vi "PathPlanner_Cmd_FindFollowHolonomicPathSimpleExecute.vi"(5 "PathPlanner_Cmd_FollowHolConfig":T13={"HOLONOMIC_CTRL_PACK_TUNING"={"X PID Tuning"={"Kp"=0.0, "Ki"=0.0, "Kd"=0.0, "MaximumIntegral"=9.9e+30, "MinimumIntegral"=-9.9e+30, "IntegralZone"=9.9e+30}, "Y PID Tuning"={"Kp"=0.0, "Ki"=0.0, "Kd"=0.0, "MaximumIntegral"=9.9e+30, "MinimumIntegral"=-9.9e+30, "IntegralZone"=9.9e+30}, "thetaProfiledPID_CTRL"={"Controller"={"Kp"=0.0, "Ki"=0.0, "Kd"=0.0, "Period"=0.0, "Max_Integral"=1.0, "Min_Integral"=-1.0, "Max_Input"=0.0, "Min_Input"=0.0, "Continuous"=FALSE, "PositionError"=0.0, "VelocityError"=0.0, "PrevError"=0.0, "Total_Integral"=0.0, "PositionTolerance"=0.05, "VelocityTolerance"=9.99e+35, "SetPoint"=0.0, "Kf"=0.0, "Prev_Deriv"=0.0, "Prev_Deriv 2"=0.0, "DerivativeFilter"=FALSE, "Min_Output"=-9.99e+35, "Max_Output"=9.9e+35, "Prev_F_P"=0.0, "Prev_F_P_2"=0.0, "AntiWindupActive"=FALSE, "Measurement"=0.0, "IntegralZone"=9.9e+30}, "Goal"={"Position"=0.0, "Velocity"=0.0}, "Setpoint"={"Position"=0.0, "Velocity"=0.0}, "Constraint"={"MaxVelocity"=0.0, "MaxAcceleration"=0.0}}}, "Max Wheel Speed M/S"=0.0, "Tolerance SI"={"TRANSLATION"={"X"=0.04, "Y"=0.04}, "ROTATION"={"VALUE"=0.034906585039887, "COS"=0.999390827019096, "SIN"=0.034899496702501}}, "Drive Base Radius M"=0.0, "ControlPastEnd_Sec"=3.0, "ReplanningConfig"={"enableInitialReplanning"=FALSE, "enableDynamicReplanning"=FALSE, "dynamicReplanningTotalErrorThreshold"=0.0, "dynamicReplanningErrorSpikeThreshold"=0.0}, "Period_Sec"=0.02, "Trigger Events"=TRUE} {"Tolerance SI"."ROTATION"."SIN" format="%13.4f"; "Tolerance SI"."ROTATION"."COS" format="%13.4f"; "Tolerance SI"."ROTATION"."VALUE" format="%13.4f"; "Tolerance SI"."TRANSLATION"."Y" format="%14.3f"; "Tolerance SI"."TRANSLATION"."X" format="%14.3f"; "HOLONOMIC_CTRL_PACK_TUNING"."thetaProfiledPID_CTRL"."Constraint"."MaxAcceleration" format="%16_6e"; "HOLONOMIC_CTRL_PACK_TUNING"."thetaProfiledPID_CTRL"."Constraint"."MaxVelocity" format="%16_6e"; "HOLONOMIC_CTRL_PACK_TUNING"."thetaProfiledPID_CTRL"."Setpoint"."Velocity" format="%16_6e"; "HOLONOMIC_CTRL_PACK_TUNING"."thetaProfiledPID_CTRL"."Setpoint"."Position" format="%16_6e"; "HOLONOMIC_CTRL_PACK_TUNING"."thetaProfiledPID_CTRL"."Goal"."Velocity" format="%16_6e"; "HOLONOMIC_CTRL_PACK_TUNING"."thetaProfiledPID_CTRL"."Goal"."Position" format="%16_6e"; "HOLONOMIC_CTRL_PACK_TUNING"."thetaProfiledPID_CTRL"."Controller"."IntegralZone" format="%16_6e"; "HOLONOMIC_CTRL_PACK_TUNING"."thetaProfiledPID_CTRL"."Controller"."Measurement" format="%16_6e"; "HOLONOMIC_CTRL_PACK_TUNING"."thetaProfiledPID_CTRL"."Controller"."Prev_F_P_2" format="%16_6e"; "HOLONOMIC_CTRL_PACK_TUNING"."thetaProfiledPID_CTRL"."Controller"."Prev_F_P" format="%16_6e"; "HOLONOMIC_CTRL_PACK_TUNING"."thetaProfiledPID_CTRL"."Controller"."Max_Output" format="%16_6e"; "HOLONOMIC_CTRL_PACK_TUNING"."thetaProfiledPID_CTRL"."Controller"."Min_Output" format="%16_6e"; "HOLONOMIC_CTRL_PACK_TUNING"."thetaProfiledPID_CTRL"."Controller"."Prev_Deriv 2" format="%16_6e"; "HOLONOMIC_CTRL_PACK_TUNING"."thetaProfiledPID_CTRL"."Controller"."Prev_Deriv" format="%16_6e"; "HOLONOMIC_CTRL_PACK_TUNING"."thetaProfiledPID_CTRL"."Controller"."Kf" format="%16_6e"; "HOLONOMIC_CTRL_PACK_TUNING"."thetaProfiledPID_CTRL"."Controller"."SetPoint" format="%16_6e"; "HOLONOMIC_CTRL_PACK_TUNING"."thetaProfiledPID_CTRL"."Controller"."VelocityTolerance" format="%16_6e"; "HOLONOMIC_CTRL_PACK_TUNING"."thetaProfiledPID_CTRL"."Controller"."PositionTolerance" format="%16_6e"; "HOLONOMIC_CTRL_PACK_TUNING"."thetaProfiledPID_CTRL"."Controller"."Total_Integral" format="%16_6e"; "HOLONOMIC_CTRL_PACK_TUNING"."thetaProfiledPID_CTRL"."Controller"."PrevError" format="%16_6e"; "HOLONOMIC_CTRL_PACK_TUNING"."thetaProfiledPID_CTRL"."Controller"."VelocityError" format="%16_6e"; "HOLONOMIC_CTRL_PACK_TUNING"."thetaProfiledPID_CTRL"."Controller"."PositionError" format="%16_6e"; "HOLONOMIC_CTRL_PACK_TUNING"."thetaProfiledPID_CTRL"."Controller"."Min_Input" format="%16_6e"; "HOLONOMIC_CTRL_PACK_TUNING"."thetaProfiledPID_CTRL"."Controller"."Max_Input" format="%16_6e"; "HOLONOMIC_CTRL_PACK_TUNING"."thetaProfiledPID_CTRL"."Controller"."Min_Integral" format="%16_6e"; "HOLONOMIC_CTRL_PACK_TUNING"."thetaProfiledPID_CTRL"."Controller"."Max_Integral" format="%16_6e"; "HOLONOMIC_CTRL_PACK_TUNING"."thetaProfiledPID_CTRL"."Controller"."Period" format="%16_6e"; "HOLONOMIC_CTRL_PACK_TUNING"."thetaProfiledPID_CTRL"."Controller"."Kd" format="%16_6e"; "HOLONOMIC_CTRL_PACK_TUNING"."thetaProfiledPID_CTRL"."Controller"."Ki" format="%16_6e"; "HOLONOMIC_CTRL_PACK_TUNING"."thetaProfiledPID_CTRL"."Controller"."Kp" format="%16_6e"}, 6 "PassthroughTime_SEC":dbl=-1.0, 7 "PathPlanner_Cmd_FindConfig":T1={"Goal Position"={"X"=0.0, "Y"=0.0}, "GoalEndState"={"VelocityMPS"=0.0, "Rotation"={"VALUE"=0.0, "COS"=1.0, "SIN"=0.0}}, "PathPlannerPathConstraints"={"MaxVelocityMps;"=0.0, "MaxAccelerationMpsSq;"=0.0, "MaxAngularVelRadPsEc;"=0.0, "MaxAngularAccRadPSecSq"=0.0, "Exists"=FALSE, "Unlimited"=FALSE, "NominalVoltageVolts"=12.0}, "Rotation Delay Distance M"=0.0} {"GoalEndState"."Rotation"."SIN" format="%13.4f"; "GoalEndState"."Rotation"."COS" format="%13.4f"; "GoalEndState"."Rotation"."VALUE" format="%13.4f"; "Goal Position"."Y" step=0.25 format="%14.3f"; "Goal Position"."X" format="%14.3f"}, 8 "Enabled":bool=TRUE, 9 "Reset":bool, 10 "CurrentChassisSpeeds":T6 {"vOmega" format="%10.3f"; "vY" format="%10.3f"; "vX" format="%10.3f"}, 11 "Current Pose SI":T8={"TRANSLATION"={"X"=0.0, "Y"=0.0}, "ROTATION"={"VALUE"=0.0, "COS"=1.0, "SIN"=0.0}} {"ROTATION"."SIN" format="%13.4f"; "ROTATION"."COS" format="%13.4f"; "ROTATION"."VALUE" format="%13.4f"; "TRANSLATION"."Y" format="%14.3f"; "TRANSLATION"."X" format="%14.3f"}) -> (0 "Position Error M":dbl, 1 "Complete":bool, 2 "At Reference":bool, 3 "calcChassisSpeed":T6 {"vOmega" format="%10.3f"; "vY" format="%10.3f"; "vX" format="%10.3f"}, 4 "outHOLONOMIC_DRV_CTRL":T7={"poseTolerance"={"TRANSLATION"={"X"=0.0, "Y"=0.0}, "ROTATION"={"VALUE"=0.0, "COS"=1.0, "SIN"=0.0}}, "poseError"={"TRANSLATION"={"X"=0.0, "Y"=0.0}, "ROTATION"={"VALUE"=0.0, "COS"=1.0, "SIN"=0.0}}, "Enabled"=TRUE, "PID_xCtrl"={"Kp"=0.0, "Ki"=0.0, "Kd"=0.0, "Period"=0.0, "Max_Integral"=1.0, "Min_Integral"=-1.0, "Max_Input"=0.0, "Min_Input"=0.0, "Continuous"=FALSE, "PositionError"=0.0, "VelocityError"=0.0, "PrevError"=0.0, "Total_Integral"=0.0, "PositionTolerance"=0.05, "VelocityTolerance"=9.99e+35, "SetPoint"=0.0, "Kf"=0.0, "Prev_Deriv"=0.0, "Prev_Deriv 2"=0.0, "DerivativeFilter"=FALSE, "Min_Output"=-9.99e+35, "Max_Output"=9.9e+35, "Prev_F_P"=0.0, "Prev_F_P_2"=0.0, "AntiWindupActive"=FALSE, "Measurement"=0.0, "IntegralZone"=9.9e+30}, "PID_yCtrl"={"Kp"=0.0, "Ki"=0.0, "Kd"=0.0, "Period"=0.0, "Max_Integral"=1.0, "Min_Integral"=-1.0, "Max_Input"=0.0, "Min_Input"=0.0, "Continuous"=FALSE, "PositionError"=0.0, "VelocityError"=0.0, "PrevError"=0.0, "Total_Integral"=0.0, "PositionTolerance"=0.05, "VelocityTolerance"=9.99e+35, "SetPoint"=0.0, "Kf"=0.0, "Prev_Deriv"=0.0, "Prev_Deriv 2"=0.0, "DerivativeFilter"=FALSE, "Min_Output"=-9.99e+35, "Max_Output"=9.9e+35, "Prev_F_P"=0.0, "Prev_F_P_2"=0.0, "AntiWindupActive"=FALSE, "Measurement"=0.0, "IntegralZone"=9.9e+30}, "PROF_PID_thetaCtrl"={"Controller"={"Kp"=0.0, "Ki"=0.0, "Kd"=0.0, "Period"=0.0, "Max_Integral"=1.0, "Min_Integral"=-1.0, "Max_Input"=0.0, "Min_Input"=0.0, "Continuous"=FALSE, "PositionError"=0.0, "VelocityError"=0.0, "PrevError"=0.0, "Total_Integral"=0.0, "PositionTolerance"=0.05, "VelocityTolerance"=9.99e+35, "SetPoint"=0.0, "Kf"=0.0, "Prev_Deriv"=0.0, "Prev_Deriv 2"=0.0, "DerivativeFilter"=FALSE, "Min_Output"=-9.99e+35, "Max_Output"=9.9e+35, "Prev_F_P"=0.0, "Prev_F_P_2"=0.0, "AntiWindupActive"=FALSE, "Measurement"=0.0, "IntegralZone"=9.9e+30}, "Goal"={"Position"=0.0, "Velocity"=0.0}, "Setpoint"={"Position"=0.0, "Velocity"=0.0}, "Constraint"={"MaxVelocity"=0.0, "MaxAcceleration"=0.0}}, "RotationError"={"VALUE"=0.0, "COS"=1.0, "SIN"=0.0}, "FirstRun"=TRUE} {"RotationError"."SIN" format="%13.4f"; "RotationError"."COS" format="%13.4f"; "RotationError"."VALUE" format="%13.4f"; "PROF_PID_thetaCtrl"."Constraint"."MaxAcceleration" format="%16_6e"; "PROF_PID_thetaCtrl"."Constraint"."MaxVelocity" format="%16_6e"; "PROF_PID_thetaCtrl"."Setpoint"."Velocity" format="%16_6e"; "PROF_PID_thetaCtrl"."Setpoint"."Position" format="%16_6e"; "PROF_PID_thetaCtrl"."Goal"."Velocity" format="%16_6e"; "PROF_PID_thetaCtrl"."Goal"."Position" format="%16_6e"; "PROF_PID_thetaCtrl"."Controller"."IntegralZone" format="%16_6e"; "PROF_PID_thetaCtrl"."Controller"."Measurement" format="%16_6e"; "PROF_PID_thetaCtrl"."Controller"."Prev_F_P_2" format="%16_6e"; "PROF_PID_thetaCtrl"."Controller"."Prev_F_P" format="%16_6e"; "PROF_PID_thetaCtrl"."Controller"."Max_Output" format="%16_6e"; "PROF_PID_thetaCtrl"."Controller"."Min_Output" format="%16_6e"; "PROF_PID_thetaCtrl"."Controller"."Prev_Deriv 2" format="%16_6e"; "PROF_PID_thetaCtrl"."Controller"."Prev_Deriv" format="%16_6e"; "PROF_PID_thetaCtrl"."Controller"."Kf" format="%16_6e"; "PROF_PID_thetaCtrl"."Controller"."SetPoint" format="%16_6e"; "PROF_PID_thetaCtrl"."Controller"."VelocityTolerance" format="%16_6e"; "PROF_PID_thetaCtrl"."Controller"."PositionTolerance" format="%16_6e"; "PROF_PID_thetaCtrl"."Controller"."Total_Integral" format="%16_6e"; "PROF_PID_thetaCtrl"."Controller"."PrevError" format="%16_6e"; "PROF_PID_thetaCtrl"."Controller"."VelocityError" format="%16_6e"; "PROF_PID_thetaCtrl"."Controller"."PositionError" format="%16_6e"; "PROF_PID_thetaCtrl"."Controller"."Min_Input" format="%16_6e"; "PROF_PID_thetaCtrl"."Controller"."Max_Input" format="%16_6e"; "PROF_PID_thetaCtrl"."Controller"."Min_Integral" format="%16_6e"; "PROF_PID_thetaCtrl"."Controller"."Max_Integral" format="%16_6e"; "PROF_PID_thetaCtrl"."Controller"."Period" format="%16_6e"; "PROF_PID_thetaCtrl"."Controller"."Kd" format="%16_6e"; "PROF_PID_thetaCtrl"."Controller"."Ki" format="%16_6e"; "PROF_PID_thetaCtrl"."Controller"."Kp" format="%16_6e"; "PID_yCtrl"."IntegralZone" format="%16_6e"; "PID_yCtrl"."Measurement" format="%16_6e"; "PID_yCtrl"."Prev_F_P_2" format="%16_6e"; "PID_yCtrl"."Prev_F_P" format="%16_6e"; "PID_yCtrl"."Max_Output" format="%16_6e"; "PID_yCtrl"."Min_Output" format="%16_6e"; "PID_yCtrl"."Prev_Deriv 2" format="%16_6e"; "PID_yCtrl"."Prev_Deriv" format="%16_6e"; "PID_yCtrl"."Kf" format="%16_6e"; "PID_yCtrl"."SetPoint" format="%16_6e"; "PID_yCtrl"."VelocityTolerance" format="%16_6e"; "PID_yCtrl"."PositionTolerance" format="%16_6e"; "PID_yCtrl"."Total_Integral" format="%16_6e"; "PID_yCtrl"."PrevError" format="%16_6e"; "PID_yCtrl"."VelocityError" format="%16_6e"; "PID_yCtrl"."PositionError" format="%16_6e"; "PID_yCtrl"."Min_Input" format="%16_6e"; "PID_yCtrl"."Max_Input" format="%16_6e"; "PID_yCtrl"."Min_Integral" format="%16_6e"; "PID_yCtrl"."Max_Integral" format="%16_6e"; "PID_yCtrl"."Period" format="%16_6e"; "PID_yCtrl"."Kd" format="%16_6e"; "PID_yCtrl"."Ki" format="%16_6e"; "PID_yCtrl"."Kp" format="%16_6e"; "PID_xCtrl"."IntegralZone" format="%16_6e"; "PID_xCtrl"."Measurement" format="%16_6e"; "PID_xCtrl"."Prev_F_P_2" format="%16_6e"; "PID_xCtrl"."Prev_F_P" format="%16_6e"; "PID_xCtrl"."Max_Output" format="%16_6e"; "PID_xCtrl"."Min_Output" format="%16_6e"; "PID_xCtrl"."Prev_Deriv 2" format="%16_6e"; "PID_xCtrl"."Prev_Deriv" format="%16_6e"; "PID_xCtrl"."Kf" format="%16_6e"; "PID_xCtrl"."SetPoint" format="%16_6e"; "PID_xCtrl"."VelocityTolerance" format="%16_6e"; "PID_xCtrl"."PositionTolerance" format="%16_6e"; "PID_xCtrl"."Total_Integral" format="%16_6e"; "PID_xCtrl"."PrevError" format="%16_6e"; "PID_xCtrl"."VelocityError" format="%16_6e"; "PID_xCtrl"."PositionError" format="%16_6e"; "PID_xCtrl"."Min_Input" format="%16_6e"; "PID_xCtrl"."Max_Input" format="%16_6e"; "PID_xCtrl"."Min_Integral" format="%16_6e"; "PID_xCtrl"."Max_Integral" format="%16_6e"; "PID_xCtrl"."Period" format="%16_6e"; "PID_xCtrl"."Kd" format="%16_6e"; "PID_xCtrl"."Ki" format="%16_6e"; "PID_xCtrl"."Kp" format="%16_6e"; "poseError"."ROTATION"."SIN" format="%13.4f"; "poseError"."ROTATION"."COS" format="%13.4f"; "poseError"."ROTATION"."VALUE" format="%13.4f"; "poseError"."TRANSLATION"."Y" format="%14.3f"; "poseError"."TRANSLATION"."X" format="%14.3f"; "poseTolerance"."ROTATION"."SIN" format="%13.4f"; "poseTolerance"."ROTATION"."COS" format="%13.4f"; "poseTolerance"."ROTATION"."VALUE" format="%13.4f"; "poseTolerance"."TRANSLATION"."Y" format="%14.3f"; "poseTolerance"."TRANSLATION"."X" format="%14.3f"})   [LabVIEW 2019, in "PathPlanner24.lvlib"]
doc: "DOCUMENTATION IS NOT COMPLETE.\n\nFind and follow a path for holonomic (swerve and mecanum) drive robots using holonomic controller.\n \n \nInputs:\n - CurrentPoseSi - pose2d - The current pose calculated by odometry or pose estimation. The pose can be absolute or relative depending on what type of trajectory is being followed.\n - Reset - boolean - When TRUE the holonomic drive controller is reset. This should be set to TRUE for the first execution of a trajectory.\n - Enabled - boolean - When TRUE, closed loop control is enabled. (Optional. Default: TRUE)\n - Period - double - The loop period in seconds for this controller. (Optional. Default: 0.020)\n\nOutputs:\n - CalcChassisSpeed - cluster - The desired chassis speed in SI units.\n - AtReference - boolean - TRUE if the robots position is within the defined tolerance.\n - PositionError - pose2d - Position error in SI units. How far the robot is away from the desired trajectory position.\n - out_Holonomic_Drive_Ctrl - THe current holonomic drive controller data cluster. This is mainly for diagnostic purposes."
uses:
  PathPlanner24.lvlib
  <vilib>/Rock Robotics/WPI/ThirdParty/JAS_Junk/TrajLib/TypeDef/POSE2D.ctl
  <vilib>/Rock Robotics/WPI/ThirdParty/JAS_Junk/TrajLib/TypeDef/TRANSLATION2D.ctl
  <vilib>/Rock Robotics/WPI/ThirdParty/JAS_Junk/TrajLib/TypeDef/ROTATION2D.ctl
  TypeDef/PathPlannerCmdFollowHolConfig.ctl
  <vilib>/Rock Robotics/WPI/ThirdParty/JAS_Junk/TrajLib/TypeDef/HOLONOMIC_PACK_TUNING.ctl
  <vilib>/Rock Robotics/WPI/ThirdParty/JAS_Junk/TrajLib/TypeDef/PID_TUNING.ctl
  <vilib>/Rock Robotics/WPI/ThirdParty/JAS_Junk/TrajLib/TypeDef/PROFILED_PID_CONTROLLER.ctl
  <vilib>/Rock Robotics/WPI/ThirdParty/JAS_Junk/TrajLib/TypeDef/PID_CONTROLLER.ctl
  <vilib>/Rock Robotics/WPI/ThirdParty/JAS_Junk/TrajLib/TypeDef/TRAPEZOID_PROFILE_STATE.ctl
  <vilib>/Rock Robotics/WPI/ThirdParty/JAS_Junk/TrajLib/TypeDef/TRAPEZOID_PROFILE_CONSTRAINT.ctl
  TypeDef/PathPlannerReplanningConfig.ctl
  <vilib>/Rock Robotics/WPI/ThirdParty/JAS_Junk/TrajLib/TypeDef/HOLONOMIC_DRV_CTRL.ctl
  <vilib>/Rock Robotics/WPI/ThirdParty/JAS_Junk/TrajLib/TypeDef/CHASSIS_SPEEDS.ctl
  TypeDef/PathPlannerCmdFindConfig.ctl
  TypeDef/PathPlannerGoalEndState.ctl
  TypeDef/PathPlannerPathConstraints.ctl
  <vilib>/Rock Robotics/WPI/ThirdParty/JAS_Junk/TrajLib/Util_CalcDist.vi
  <vilib>/Rock Robotics/WPI/ThirdParty/JAS_Junk/TrajLib/Trajectory_Library.lvlib
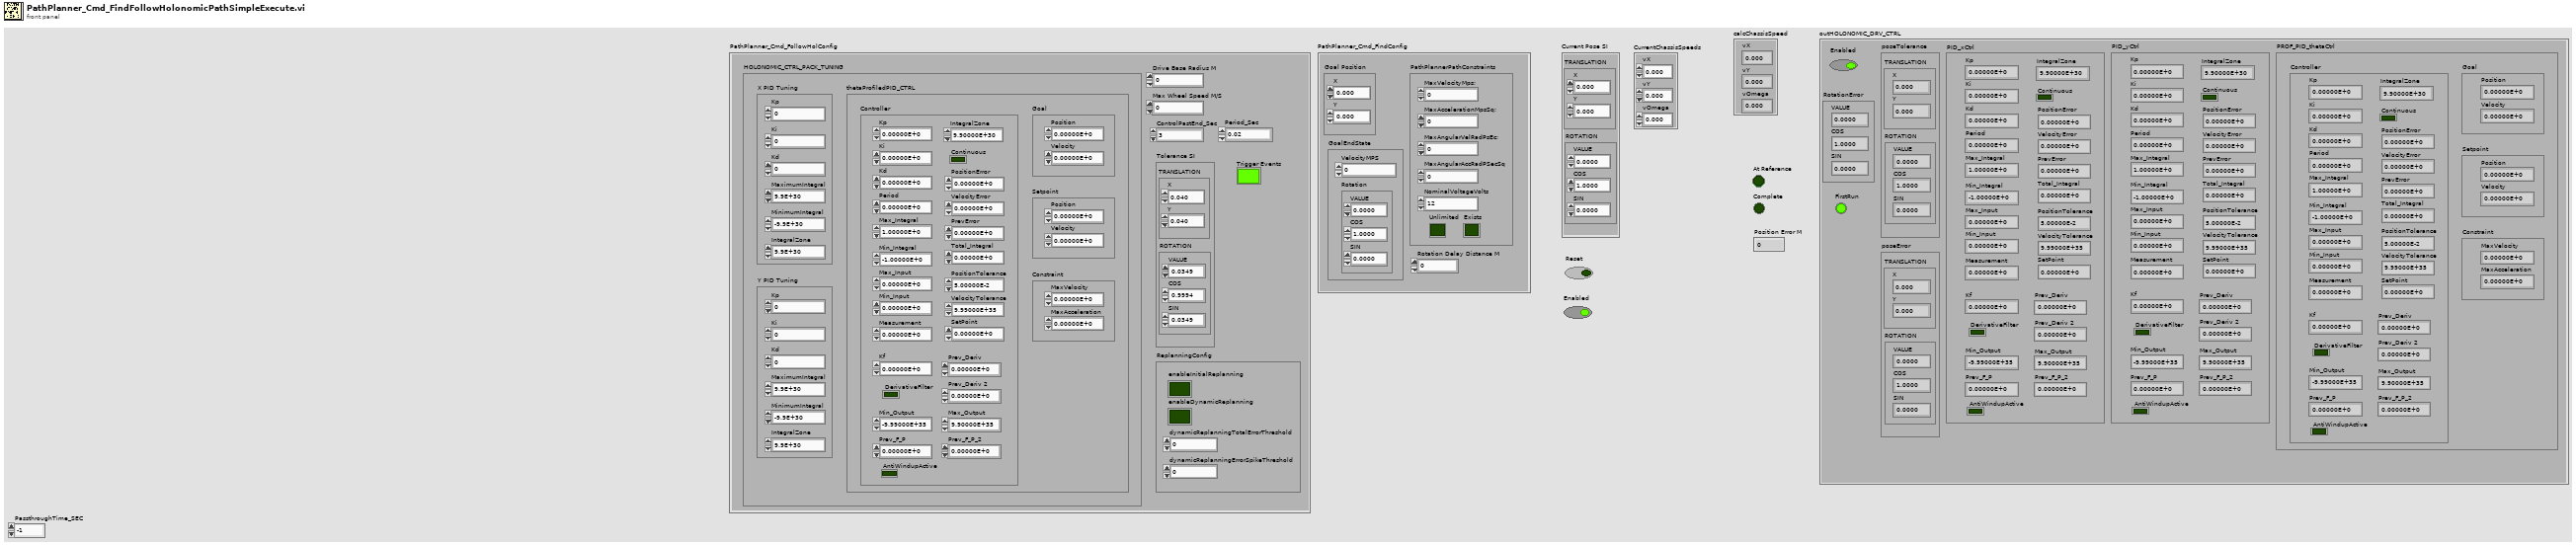
[diagram p1: front panel]
types:
  T1 = typedef "PathPlanner24.lvlib/PathPlannerCmdFindConfig.ctl" = cluster{"Goal Position":T2, "GoalEndState":T3, "PathPlannerPathConstraints":T5, "Rotation Delay Distance M":dbl}
  T2 = typedef "Trajectory_Library.lvlib/TRANSLATION2D.ctl" = cluster{"X":dbl, "Y":dbl}
  T3 = typedef "PathPlanner24.lvlib/PathPlannerGoalEndState.ctl" = cluster{"VelocityMPS":dbl, "Rotation":T4}
  T4 = typedef "Trajectory_Library.lvlib/ROTATION2D.ctl" = cluster{"VALUE":dbl, "COS":dbl, "SIN":dbl}
  T5 = typedef "PathPlanner24.lvlib/PathPlannerPathConstraints.ctl" = cluster{"MaxVelocityMps;":dbl, "MaxAccelerationMpsSq;":dbl, "MaxAngularVelRadPsEc;":dbl, "MaxAngularAccRadPSecSq":dbl, "Exists":bool, "Unlimited":bool, "NominalVoltageVolts":dbl}
  T6 = typedef "Trajectory_Library.lvlib/CHASSIS_SPEEDS.ctl" = cluster{"vX":dbl, "vY":dbl, "vOmega":dbl}
  T7 = typedef "Trajectory_Library.lvlib/HOLONOMIC_DRV_CTRL.ctl" = cluster{"poseTolerance":T8, "poseError":T8, "Enabled":bool, "PID_xCtrl":T9, "PID_yCtrl":T9, "PROF_PID_thetaCtrl":T10, "RotationError":T4, "FirstRun":bool}
  T8 = typedef "Trajectory_Library.lvlib/POSE2D.ctl" = cluster{"TRANSLATION":T2, "ROTATION":T4}
  T9 = typedef "Trajectory_Library.lvlib/PID_CONTROLLER.ctl" = cluster{"Kp":dbl, "Ki":dbl, "Kd":dbl, "Period":dbl, "Max_Integral":dbl, "Min_Integral":dbl, "Max_Input":dbl, "Min_Input":dbl, "Continuous":bool, "PositionError":dbl, "VelocityError":dbl, "PrevError":dbl, "Total_Integral":dbl, "PositionTolerance":dbl, "VelocityTolerance":dbl, "SetPoint":dbl, "Kf":dbl, "Prev_Deriv":dbl, "Prev_Deriv 2":dbl, "DerivativeFilter":bool, "Min_Output":dbl, "Max_Output":dbl, "Prev_F_P":dbl, "Prev_F_P_2":dbl, "AntiWindupActive":bool, "Measurement":dbl, "IntegralZone":dbl}
  T10 = typedef "Trajectory_Library.lvlib/PROFILED_PID_CONTROLLER.ctl" = cluster{"Controller":T9, "Goal":T11, "Setpoint":T11, "Constraint":T12}
  T11 = typedef "Trajectory_Library.lvlib/TRAPEZOID_PROFILE_STATE.ctl" = cluster{"Position":dbl, "Velocity":dbl}
  T12 = typedef "Trajectory_Library.lvlib/TRAPEZOID_PROFILE_CONSTRAINT.ctl" = cluster{"MaxVelocity":dbl, "MaxAcceleration":dbl}
  T13 = typedef "PathPlanner24.lvlib/PathPlannerCmdFollowHolConfig.ctl" = cluster{"HOLONOMIC_CTRL_PACK_TUNING":T14, "Max Wheel Speed M/S":dbl, "Tolerance SI":T8, "Drive Base Radius M":dbl, "ControlPastEnd_Sec":dbl, "ReplanningConfig":T16, "Period_Sec":dbl, "Trigger Events":bool}
  T14 = typedef "Trajectory_Library.lvlib/HOLONOMIC_PACK_TUNING.ctl" = cluster{"X PID Tuning":T15, "Y PID Tuning":T15, "thetaProfiledPID_CTRL":T10}
  T15 = typedef "Trajectory_Library.lvlib/PID_TUNING.ctl" = cluster{"Kp":dbl, "Ki":dbl, "Kd":dbl, "MaximumIntegral":dbl, "MinimumIntegral":dbl, "IntegralZone":dbl}
  T16 = typedef "PathPlanner24.lvlib/PathPlannerReplanningConfig.ctl" = cluster{"enableInitialReplanning":bool, "enableDynamicReplanning":bool, "dynamicReplanningTotalErrorThreshold":dbl, "dynamicReplanningErrorSpikeThreshold":dbl}
  T17 = typedef "PathPlanner24.lvlib/PathPlannerPath.ctl" = cluster{"Reversed":bool, "RotationTargets":T18[], "ConstraintZones":T19[], "EventMarkers":T20[], "GlobalConstraints":T5, "GoalEndState":T3, "AllPoints":T23[], "Name":string, "Waypoints":T24[], "PointTowardsZones":T25[], "IdealStartingState":T26, "IsChoreoPath":bool, "PreventFlipping":bool}
  T18 = typedef "PathPlanner24.lvlib/PathPlannerRotationTarget.ctl" = cluster{"position":dbl, "rotation":T4, "Exists":bool}
  T19 = typedef "PathPlanner24.lvlib/PathPlannerConstraintsZone.ctl" = cluster{"minPosition":dbl, "maxPosition":dbl, "Constraints":T5, "Present":bool}
  T20 = typedef "PathPlanner24.lvlib/PathPlannerEventMarker.ctl" = cluster{"Position":dbl, "Command":T21, "TriggerName":string, "EndPosition":dbl}
  T21 = typedef "PathPlanner24.lvlib/PathPlannerCommandUtil.ctl" = cluster{"waitTime":dbl, "name":string, "pathName":string, "commands":cluster{"type":T22, "waitTime":dbl, "name":string, "pathName":string}[], "type":T22}
  T22 = typedef "PathPlanner24.lvlib/PathPlanner_CommandUtilType_ENUM.ctl" = enum16{"Unknown", "Wait", "Named", "Path", "Sequential", "Parallel", "Race", "Deadline"}
  T23 = typedef "PathPlanner24.lvlib/PathPlannerPathPoint.ctl" = cluster{"Position":T2, "DistAlongPath":dbl, "MaxV":dbl, "Constraints":T5, "RotationTarget":T18, "WaypointRelativePos":dbl}
  T24 = typedef "PathPlanner24.lvlib/PathPlannerWaypoint.ctl" = cluster{"prevControl":T2, "anchor":T2, "nextControl":T2, "PrevExists":bool, "NextExists":bool}
  T25 = typedef "PathPlanner24.lvlib/PathPlannerPointTowardsZone.ctl" = cluster{"RotationOffset":T4, "Name":string, "TargetPosition":T2, "MinPosition":dbl, "MaxPosition":dbl}
  T26 = typedef "PathPlanner24.lvlib/PathPlannerIdealStartingState.ctl" = cluster{"VelocityMPS":dbl, "Rotation":T4}
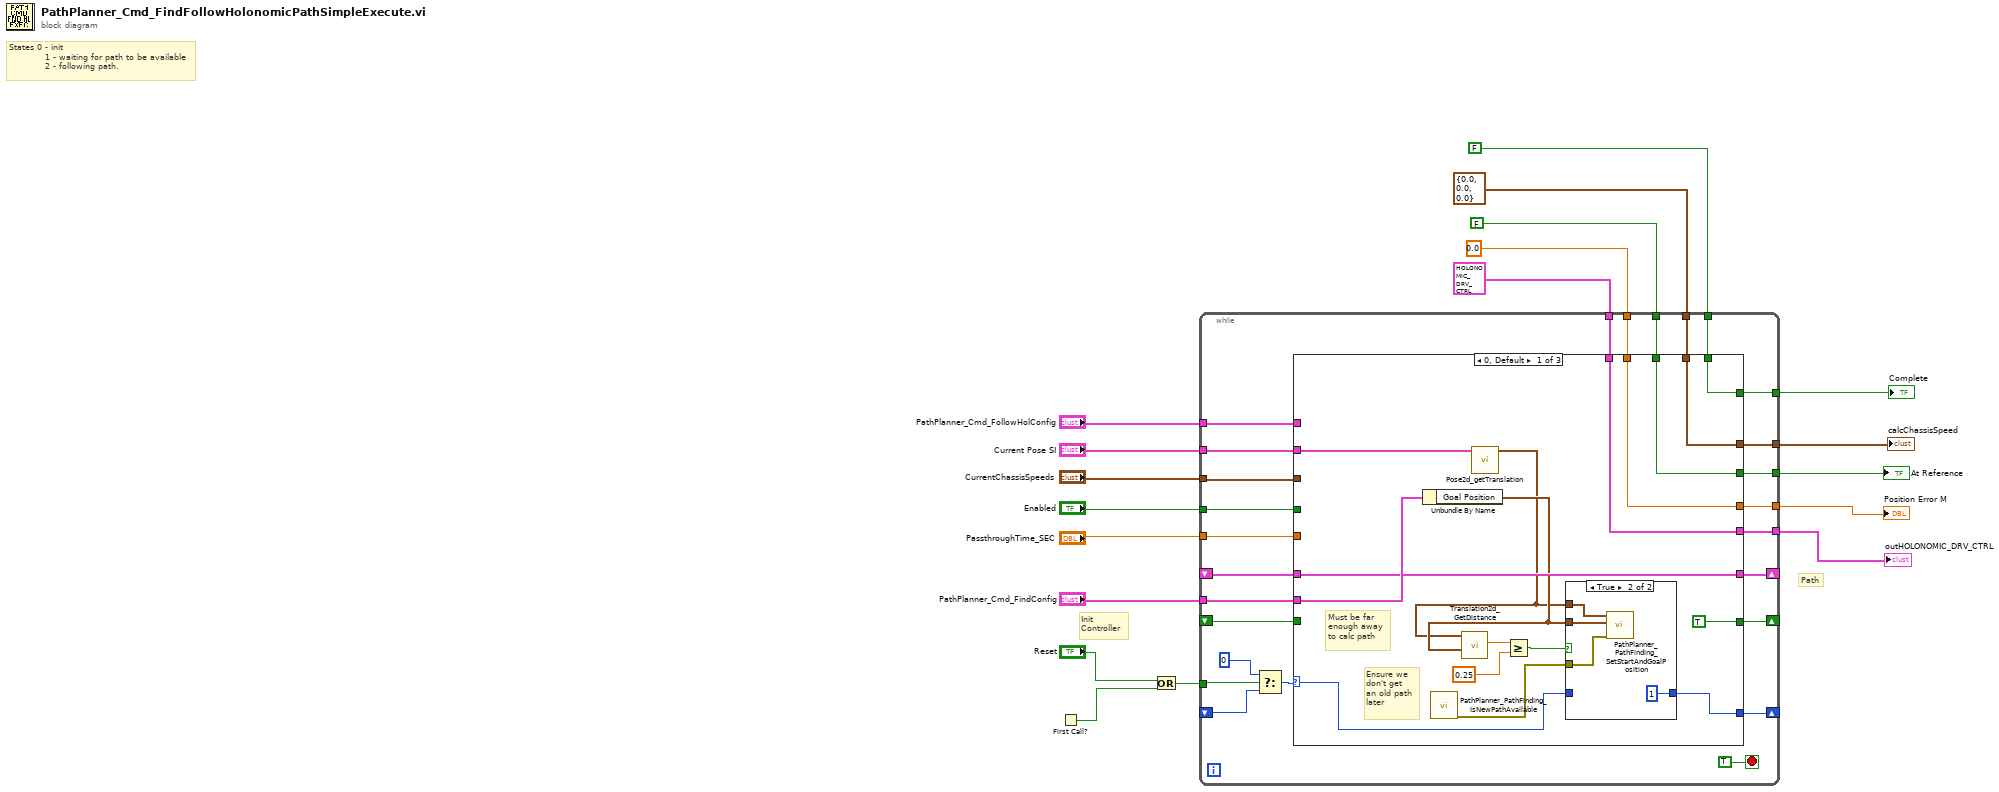
[diagram p0: block diagram]
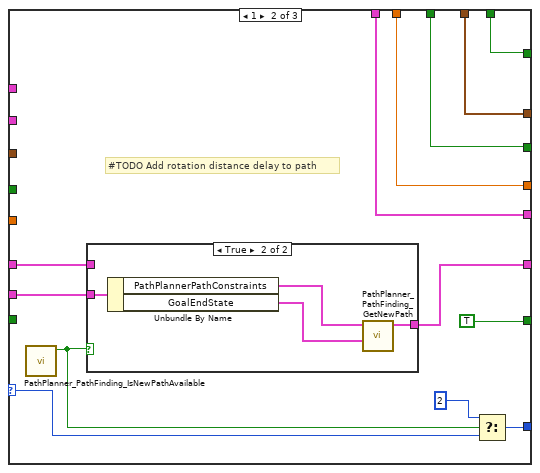
[diagram p3: hidden frame]
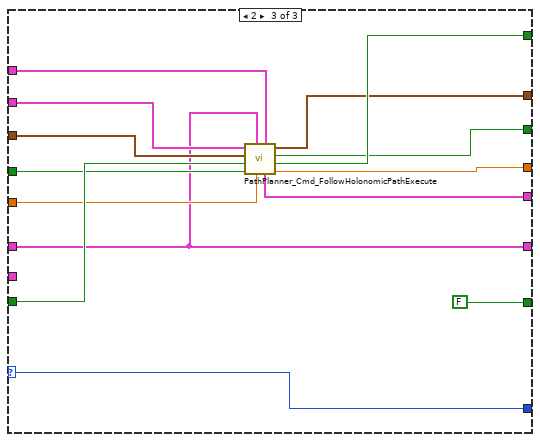
[diagram p5: hidden frame]
diagram:
  # "Init\nController"
  # "Path"
  # "States 0 - init \n            1 - waiting for path to be available\n            2 - following path."
  n1 = First Call?() -> (First Call?: T/F=w13:bool)
  n2 = Or(x="Reset", y=w13) -> (x .or. y?=w8:bool)
  n3 = while {
    tunnel: "PathPlanner_Cmd_FollowHolConfig" -> [w27]
    tunnel: "Current Pose SI" -> [w35]
    tunnel: [w45] -> w15
    tunnel: "Enabled" -> [w43]
    tunnel: [w38] -> w14
    tunnel: "CurrentChassisSpeeds" -> [w41]
    shift-right: [w36] -> _
    shift-left: _ -> [w39]
    tunnel: "PassthroughTime_SEC" -> [w40]
    tunnel: [w42] -> w11
    tunnel: [w37] -> w9
    tunnel: w8 -> [w34]
    shift-right: [w30] -> _
    shift-left: _ -> [w31]
    tunnel: "PathPlanner_Cmd_FindConfig" -> [w29]
    shift-right: [w28] -> _
    shift-left: _ -> [w26]
    tunnel: [w25] -> w6
    tunnel: T7 {"poseTolerance"={"TRANSLATION"={"X"=0.0, "Y"=0.0}, "ROTATION"={"VALUE"=0.0, "COS"=1.0, "SIN"=0.0}}, "poseError"={"TRANSLATION"={"X"=0.0, "Y"=0.0}, "ROTATION"={"VALUE"=0.0, "COS"=1.0, "SIN"=0.0}}, "Enabled"=TRUE, "PID_xCtrl"={"Kp"=0.0, "Ki"=0.0, "Kd"=0.0, "Period"=0.0, "Max_Integral"=1.0, "Min_Integral"=-1.0, "Max_Input"=0.0, "Min_Input"=0.0, "Continuous"=FALSE, "PositionError"=0.0, "VelocityError"=0.0, "PrevError"=0.0, "Total_Integral"=0.0, "PositionTolerance"=0.05, "VelocityTolerance"=9.99e+35, "SetPoint"=0.0, "Kf"=0.0, "Prev_Deriv"=0.0, "Prev_Deriv 2"=0.0, "DerivativeFilter"=FALSE, "Min_Output"=-9.99e+35, "Max_Output"=9.9e+35, "Prev_F_P"=0.0, "Prev_F_P_2"=0.0, "AntiWindupActive"=FALSE, "Measurement"=0.0, "IntegralZone"=9.9e+30}, "PID_yCtrl"={"Kp"=0.0, "Ki"=0.0, "Kd"=0.0, "Period"=0.0, "Max_Integral"=1.0, "Min_Integral"=-1.0, "Max_Input"=0.0, "Min_Input"=0.0, "Continuous"=FALSE, "PositionError"=0.0, "VelocityError"=0.0, "PrevError"=0.0, "Total_Integral"=0.0, "PositionTolerance"=0.05, "VelocityTolerance"=9.99e+35, "SetPoint"=0.0, "Kf"=0.0, "Prev_Deriv"=0.0, "Prev_Deriv 2"=0.0, "DerivativeFilter"=FALSE, "Min_Output"=-9.99e+35, "Max_Output"=9.9e+35, "Prev_F_P"=0.0, "Prev_F_P_2"=0.0, "AntiWindupActive"=FALSE, "Measurement"=0.0, "IntegralZone"=9.9e+30}, "PROF_PID_thetaCtrl"={"Controller"={"Kp"=0.0, "Ki"=0.0, "Kd"=0.0, "Period"=0.0, "Max_Integral"=1.0, "Min_Integral"=-1.0, "Max_Input"=0.0, "Min_Input"=0.0, "Continuous"=FALSE, "PositionError"=0.0, "VelocityError"=0.0, "PrevError"=0.0, "Total_Integral"=0.0, "PositionTolerance"=0.05, "VelocityTolerance"=9.99e+35, "SetPoint"=0.0, "Kf"=0.0, "Prev_Deriv"=0.0, "Prev_Deriv 2"=0.0, "DerivativeFilter"=FALSE, "Min_Output"=-9.99e+35, "Max_Output"=9.9e+35, "Prev_F_P"=0.0, "Prev_F_P_2"=0.0, "AntiWindupActive"=FALSE, "Measurement"=0.0, "IntegralZone"=9.9e+30}, "Goal"={"Position"=0.0, "Velocity"=0.0}, "Setpoint"={"Position"=0.0, "Velocity"=0.0}, "Constraint"={"MaxVelocity"=0.0, "MaxAcceleration"=0.0}}, "RotationError"={"VALUE"=0.0, "COS"=1.0, "SIN"=0.0}, "FirstRun"=TRUE} ("outHOLONOMIC_DRV_CTRL") -> [w24]
    tunnel: FALSE ("Complete") -> [w23]
    tunnel: T6 {"vX"=0.0, "vY"=0.0, "vOmega"=0.0} ("calcChassisSpeed") -> [w22]
    tunnel: FALSE ("At Reference") -> [w21]
    tunnel: 0.0 ("Position Error M") -> [w20]
    stop <- TRUE stop-if-true
    n4 = Select(t=0, s=w34, f=w31) -> (s? t:f=w32:i32)
    n5 = case shown="0, Default" w32 {
      selector: w32 -> [w46 w68 w86]
      tunnel: [w55 w72 w95] -> w45
      tunnel: w43 -> [_ _ w90]
      tunnel: [w59 w74 w96] -> w25
      tunnel: [w60 w70 w94] -> w42
      tunnel: w41 -> [_ _ w92]
      tunnel: w40 -> [_ _ w89]
      tunnel: w39 -> [w57 w76 w87]
      tunnel: [w58 w73 w97] -> w38
      tunnel: [w54 w71 w98] -> w37
      tunnel: [w57 w77 w87] -> w36
      tunnel: w35 -> [w56 _ w93]
      tunnel: [w47 w69 w86] -> w30
      tunnel: w29 -> [w62 w78 _]
      tunnel: [TRUE TRUE FALSE] -> w28
      tunnel: w27 -> [_ _ w88]
      tunnel: w26 -> [_ _ w91]
      tunnel: w20 -> [w59 w74 _]
      tunnel: w21 -> [w58 w73 _]
      tunnel: w22 -> [w55 w72 _]
      tunnel: w23 -> [w54 w71 _]
      tunnel: w24 -> [w60 w70 _]
      frame 0, Default {
        # "Must be far\nenough away\nto calc path"
        # "Ensure we\ndon't get\nan old path\nlater"
        n6 = Unbundle By Name(w62) -> ("Goal Position"=w50:T2)
        n7 = call "PathPlanner_PathFinding_IsNewPathAvailable.vi"() -> ("error out"=w49:errorcluster)  [unwired: 10 in, 1 out]
        n8 = call <vilib>:"Pose2d_getTranslation.vi"("in POSE"=w56) -> ("outTRANSLATION"=w48:T2)  [unwired: 10 in]
        n9 = call <vilib>:"Translation2d_GetDistance.vi"("other Translation"=w50, "In Translation"=w48) -> ("Distance"=w53:dbl)  [unwired: 9 in]
        n10 = Greater Or Equal?(x=w53, y=0.25) -> (x >= y?=w51:bool)
        n11 = case shown="True" w51 {
          tunnel: w50 -> [_ w67]
          tunnel: w49 -> [_ w66]
          tunnel: w48 -> [_ w65]
          tunnel: [w63 1] -> w47
          tunnel: w46 -> [w63 _]
          frame False {
          }
          frame True {
            n12 = call "PathPlanner_PathFinding_SetStartAndGoalPosition.vi"("error in (no error)"=w66, "GoalPosition"=w67, "StartPosition"=w65) -> ()  [unwired: 8 in, 1 out]
          }
        }
      }
      frame 1 {
        # "#TODO Add rotation distance delay to path"
        n13 = call "PathPlanner_PathFinding_IsNewPathAvailable.vi"() -> ("New Path Available"=w79:bool)  [unwired: 10 in, 1 out]
        n14 = case shown="True" w79 {
          tunnel: w78 -> [_ w85]
          tunnel: [w81 w83] -> w77
          tunnel: w76 -> [w81 _]
          frame False {
          }
          frame True {
            n15 = Unbundle By Name(w85) -> ("PathPlannerPathConstraints"=w82:T5, "GoalEndState"=w84:T3)
            n16 = call "PathPlanner_PathFinding_GetNewPath.vi"("GoalEndState"=w84, "PathPlannerPathConstraints"=w82) -> ("PathPlannerPath"=w83:T17)  [unwired: 8 in, 1 out]
          }
        }
        n17 = Select(t=2, s=w79, f=w68) -> (s? t:f=w69:i32)
      }
      frame 2 {
        n18 = call "PathPlanner_Cmd_FollowHolonomicPathExecute.vi"("PathPlanner_Cmd_FollowHolConfig"=w88, "PassthroughTime_SEC"=w89, "PathPlannerPath"=w87, "Enabled"=w90, "Reset"=w91, "CurrentChassisSpeeds"=w92, "Current Pose SI"=w93) -> ("Position Error M"=w96:dbl, "Complete"=w98:bool, "At Reference"=w97:bool, "calcChassisSpeed"=w95:T6, "outHOLONOMIC_DRV_CTRL"=w94:T7)
      }
    }
  }
  "At Reference" <- w14
  "Position Error M" <- w6
  "outHOLONOMIC_DRV_CTRL" <- w11
  "calcChassisSpeed" <- w15
  "Complete" <- w9
